vi "Data Manage Thread.vi"() -> ()   [LabVIEW 2016]
uses:
  <vilib>/Utility/error.llb/DialogType.ctl
  Architecture/Queue Management/ARC_Queue Create_Single.vi
  Architecture/Queue Management/ARC_Queue Valid.vi
  Architecture/Queue Management/ARC_Queue Insert Element.vi
  Architecture/Queue Management/ARC_Queue Remove Element.vi
  Architecture/Queue Management/ARC_Queue Destroy_Single.vi
panel:
  in  "Parameter":cluster{"Q-Local":string, "Variant":variant}
  out "Error Report":string
  out "Current State":string
  in  "Exit Program":bool
  in  "TempVariable":T1
  # "/* -------- Notes for All Users -------- */\nRecommand : \n[1].Display Setting Resolution -> 1440x900\n[2].Read Arch Notes First.\n[3].Make A Call When You Are In Trouble.\n\nTeam Members:\nPansino Soft,Pansino SDMA\n\nCopyright@2013 Pansino.Beijing\n\nVersion Number: 2013"
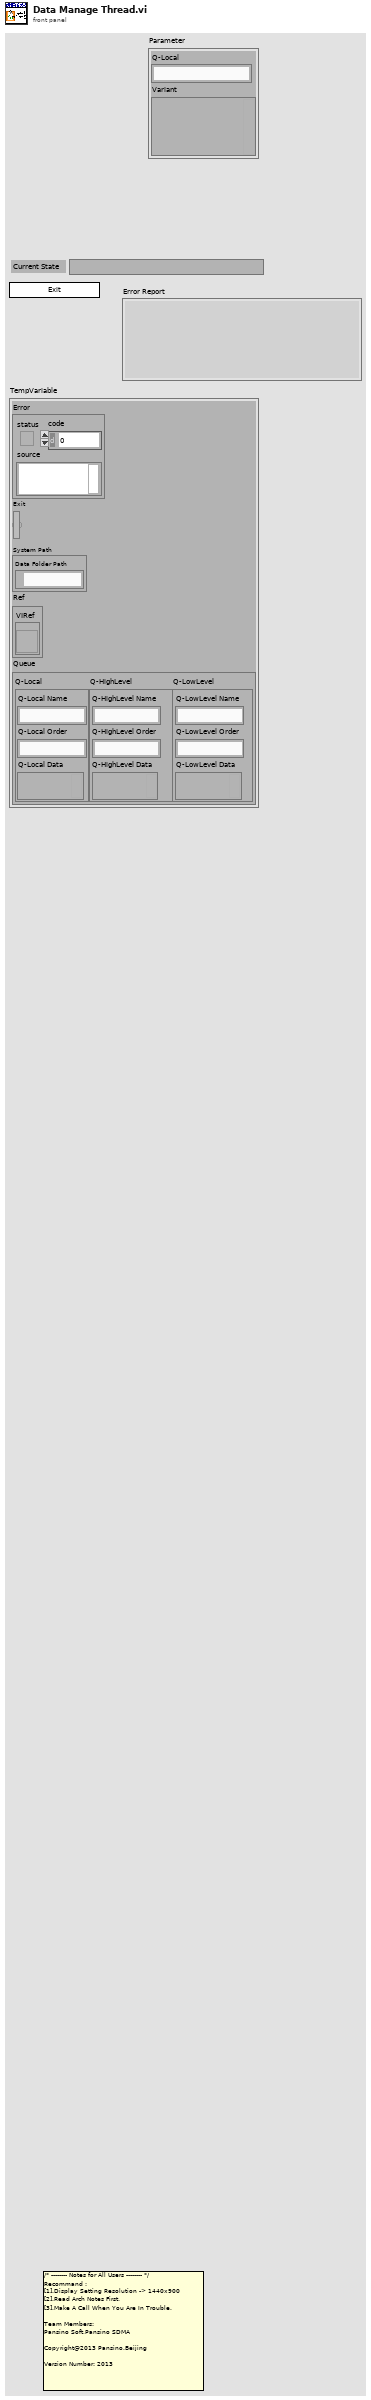
[diagram p1: front panel]
types:
  T1 = cluster{"Error":errorcluster, "Exit":bool, "System Path":cluster{"Data Folder Path":path}, "Ref":cluster{"VIRef":refnum<vi>}, "Queue":cluster{"Q-Local":cluster{"Q-Local Name":string, "Q-Local Order":string, "Q-Local Data":variant}, "Q-HighLevel":cluster{"Q-HighLevel Name":string, "Q-HighLevel Order":string, "Q-HighLevel Data":variant}, "Q-LowLevel":cluster{"Q-LowLevel Name":string, "Q-LowLevel Order":string, "Q-LowLevel Data":variant}}}
  T2 = typedef "DialogType.ctl" = u16
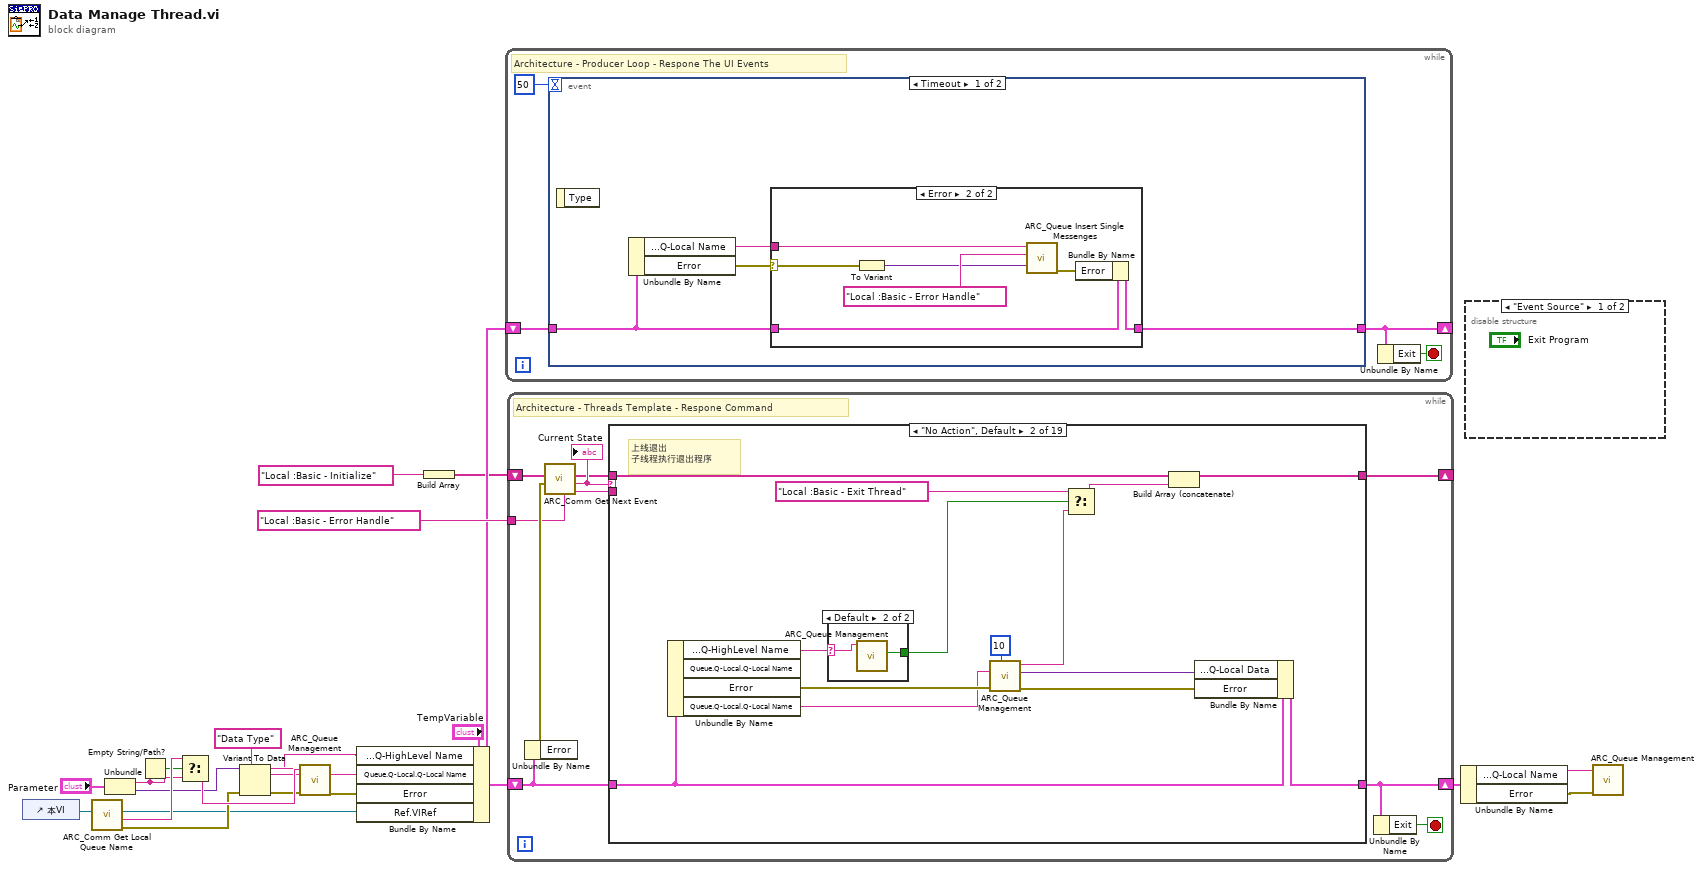
[diagram p0: block diagram]
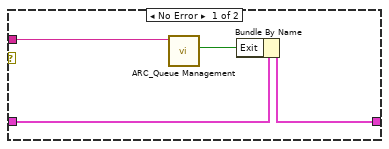
[diagram p2: hidden frame]
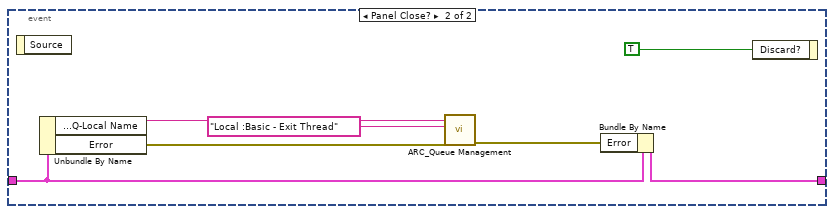
[diagram p3: hidden frame]
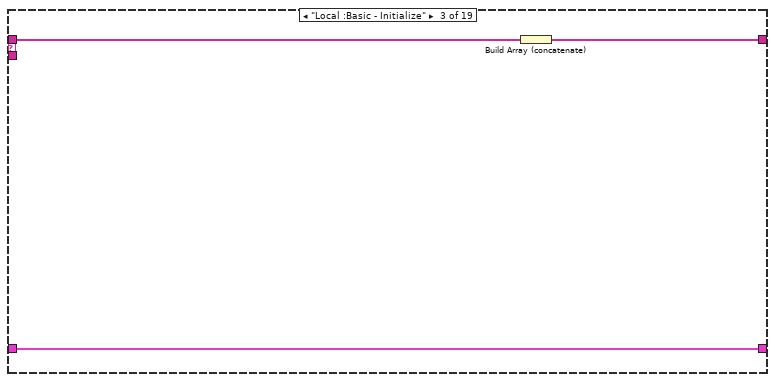
[diagram p7: hidden frame]
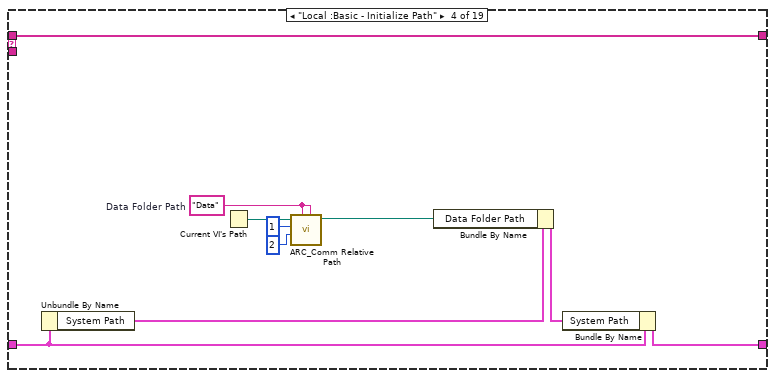
[diagram p8: hidden frame]
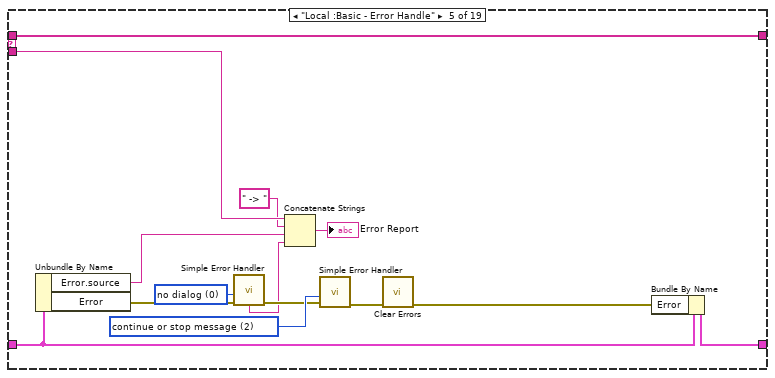
[diagram p9: hidden frame]
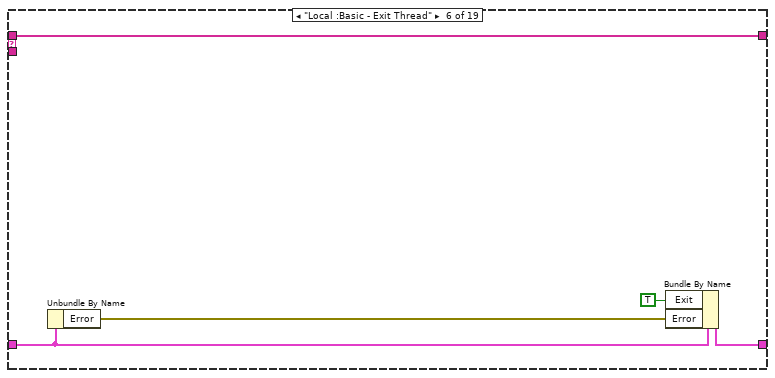
[diagram p10: hidden frame]
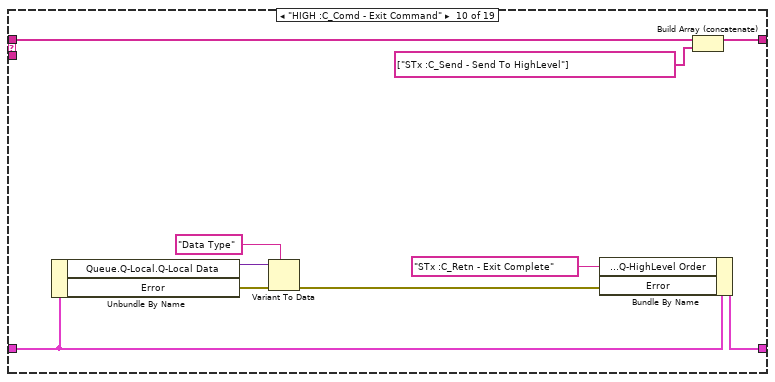
[diagram p14: hidden frame]
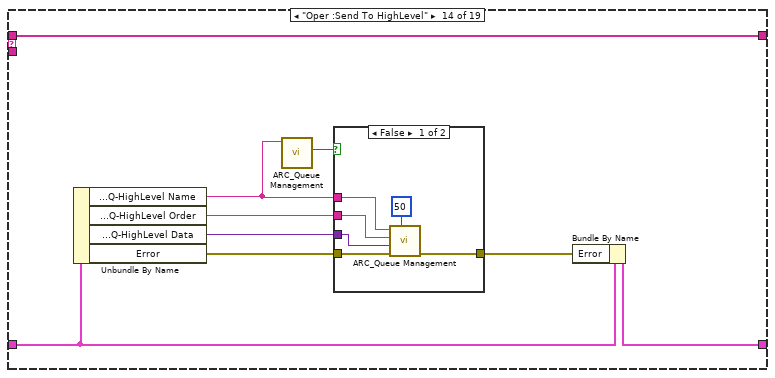
[diagram p18: hidden frame]
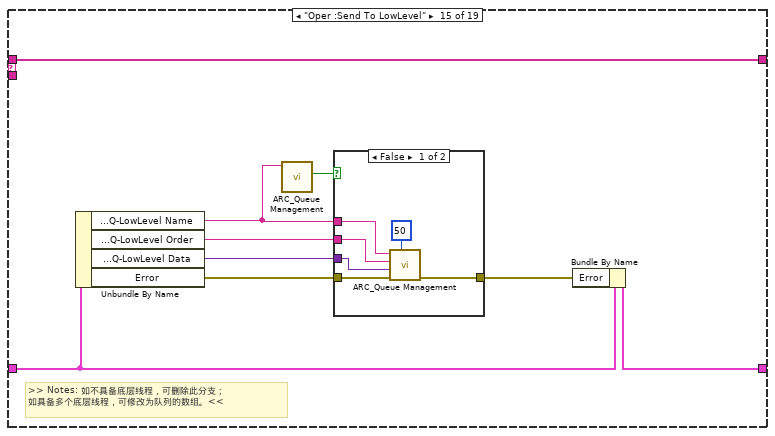
[diagram p20: hidden frame]
diagram:
  n1 = control-ref of="本VI"() -> (w7:refnum<vi>)
  n2 = call "ARC_Comm Get Local Queue Name.vi"("VI Ref"=w7) -> ("error out"=w8:errorcluster, "VI  Name"=w13:string, "VI Ref out"=w4:refnum<vi>)  [unwired: 8 in]
  n3 = Unbundle("Parameter") -> ("Q-Local"=w9:string, "Variant"=w12:variant)
  n4 = Empty String/Path?(string/path=w9) -> (empty?=w11:bool)
  n5 = Select(t=w13, s=w11, f=w9) -> (s? t:f=w14:string)
  n6 = Variant To Data(error in=w8, type="Data Type" ("Q-Command"), Variant=w12) -> (data=w1:string, error out=w6:errorcluster)
  n7 = call-poly "ARC_Queue Management.vi"("error in"=w6, "Queue Name"=w14) -> ("error out"=w3:errorcluster, "Queue Name dup"=w2:string)  [unwired: 7 in, 1 out]
  n8 = Bundle By Name(cluster="TempVariable", "Queue.Q-HighLevel.Q-HighLevel Name"=w1, "Queue.Q-Local.Q-Local Name"=w2, "Error"=w3, "Ref.VIRef"=w4) -> (w17:T1)
  n9 = Build Array("Local :Basic - Initialize") -> (w15:string[])
  n10 = while {
    shift-right: [w24] -> _
    shift-left: w17 -> [w25]
    stop <- w23 stop-if-true
    # "Architecture - Producer Loop - Respone The UI Events"
    n11 = event shown="[0] Timeout" {
      selector: _ -> [_ _]
      dyn-events: _ -> [_ _]
      timeout: 50 -> [_ _]
      tunnel: w25 -> [w29 w46]
      tunnel: [w30 w45] -> w24
      event Timeout {
        n12 = event-data() -> ()  [unwired: 1 in, 1 out]
        n13 = Unbundle By Name(w29) -> ("Queue.Q-Local.Q-Local Name"=w28:string, "Error"=w27:errorcluster)
        n14 = case shown="Error" w27 {
          selector: w27 -> [_ w41]
          tunnel: [w34 w39] -> w30
          tunnel: w29 -> [w32 w40]
          tunnel: w28 -> [w31 w38]
          frame No Error {
            n15 = call-poly "ARC_Queue Management.vi"("Queue Name(unamed)"=w31) -> ("Not Exist?"=w33:bool)  [unwired: 8 in, 2 out]
            n16 = Bundle By Name(cluster=w32, "Exit"=w33) -> (w34:T1)
          }
          frame Error {
            n17 = To Variant(anything=w41) -> (Variant=w36:variant)
            n18 = call "ARC_Queue Insert Single Messenges.vi"("Data"=w36, "Order"="Local :Basic - Error Handle" ("Event"), "Queue Name"=w38) -> ("error out"=w35:errorcluster)  [unwired: 8 in]
            n19 = Bundle By Name(cluster=w40, "Error"=w35) -> (w39:T1)
          }
        }
      }
      event Panel Close? {
        n20 = event-data() -> ()  [unwired: 1 in, 1 out]
        n21 = Unbundle By Name(w46) -> ("Queue.Q-Local.Q-Local Name"=w43:string, "Error"=w47:errorcluster)
        n22 = call-poly "ARC_Queue Management.vi"("error in (no error)"=w47, "Event"="Local :Basic - Exit Thread", "Queue Name(unamed)"=w43) -> ("error out"=w44:errorcluster)  [unwired: 7 in, 1 out]
        n23 = Bundle By Name(cluster=w46, "Error"=w44) -> (w45:T1)
        n24 = event-data("Discard?"=TRUE ("放弃？")) -> ()  [unwired: 1 in, 1 out]
      }
    }
    n25 = Unbundle By Name(w24) -> ("Exit"=w23:bool)
  }
  n26 = while {
    shift-right: [w52] -> w22
    shift-left: w17 -> [w54]
    shift-right: [w55] -> _
    shift-left: w15 -> [w58]
    tunnel: "Local :Basic - Error Handle" ("Error Handle") -> [w50]
    stop <- w51 stop-if-true
    # "Architecture - Threads Template - Respone Command"
    n27 = Unbundle By Name(w54) -> ("Error"=w53:errorcluster)
    n28 = call "ARC_Comm Get Next Event.vi"("Error Handle"=w50, "error in (no error)"=w53, "event queue in"=w58) -> ("prev event"=w49:string, "next event"=w57:string, "event queue out"=w56:string[])  [unwired: 3 in]
    "Current State" <- w57
    n29 = case shown="\"No Action\", Default" w57 {
      tunnel: w54 -> [w59 w74 w78 w87 w101 w105 w109 w111 w113 w121 w125 w127 w129 w136 w152 w163 w168 w175 w181]
      tunnel: w56 -> [w60 w67 w79 w89 w103 w108 w110 w112 w114 w124 w126 w128 w130 w139 w155 w164 w166 w176 w179]
      tunnel: [w60 w66 w77 w89 w103 w108 w110 w112 w114 w122 w126 w128 w130 w139 w155 w164 w165 w176 w178] -> w55
      tunnel: [w59 w73 w78 w88 w102 w106 w109 w111 w113 w123 w125 w127 w129 w135 w151 w163 w167 w174 w180] -> w52
      tunnel: w49 -> [_ _ _ _ w94 _ _ _ _ _ _ _ _ _ _ _ _ _ _]
      frame "----------Core Status----------" {
      }
      frame "No Action", Default {
        # "上线退出\n子线程执行退出程序"
        n30 = Unbundle By Name(w74) -> ("Queue.Q-HighLevel.Q-HighLevel Name"=w69:string, "Error"=w70:errorcluster, "Queue.Q-Local.Q-Local Name"=w68:string)  [unwired: 1 out]
        n31 = case shown="Default" w69 {
          selector: w69 -> [_ w75]
          tunnel: [_ w76] -> w64
          frame "" {
          }
          frame Default {
            n32 = call-poly "ARC_Queue Management.vi"("Queue Name(unamed)"=w75) -> ("Not Exist?"=w76:bool)  [unwired: 8 in, 2 out]
          }
        }
        n33 = call-poly "ARC_Queue Management.vi"("Time out(-1)_queue out"=10, "error in (no error)"=w70, "Queue Name(unamed)"=w68) -> ("error out"=w72:errorcluster, "Data"=w71:variant, "Event"=w62:string)  [unwired: 5 in, 1 out]
        n34 = Select(t="Local :Basic - Exit Thread" ("Event"), s=w64, f=w62) -> (s? t:f=w61:string)
        n35 = Build Array (concatenate)(w67, w61) -> (w66:string[])
        n36 = Bundle By Name(cluster=w74, "Queue.Q-Local.Q-Local Data"=w71, "Error"=w72) -> (w73:T1)
      }
      frame "Local :Basic - Initialize" {
        n37 = Build Array (concatenate)(w79) -> (w77:string[])
      }
      frame "Local :Basic - Initialize Path" {
        w82 = "Data"  # Data Folder Path
        n38 = Unbundle By Name(w87) -> ("System Path"=w81:cluster{"Data Folder Path":path})
        n39 = Current VI's Path() -> (path=w83:path)
        n40 = call "ARC_Comm Relative Path.vi"("Development Relative Path"=w82, "Run Time relative path"=w82, "Run-Time File Depth"=2, "Development File Depth"=1, "Root Path"=w83) -> ("Relative Path"=w86:path)  [unwired: 5 in, 1 out]
        n41 = Bundle By Name(cluster=w81, "Data Folder Path"=w86) -> (w80:cluster{"Data Folder Path":path})
        n42 = Bundle By Name(cluster=w87, "System Path"=w80) -> (w88:T1)
      }
      frame "Local :Basic - Error Handle" {
        w95 = T2 0 items=["no dialog", "OK message", "continue or stop message", "OK message + warnings", "continue/stop + warnings"] ("type of dialog (OK msg:1)")
        w98 = T2 2 items=["no dialog", "OK message", "continue or stop message", "OK message + warnings", "continue/stop + warnings"] ("type of dialog (OK msg:1)")
        n43 = Unbundle By Name(w101) -> ("Error.source"=w90:string, "Error"=w97:errorcluster)
        n44 = call <vilib>:"Simple Error Handler.vi"("type of dialog (OK msg:1)"=w95, "error in (no error)"=w97) -> ("error out"=w96:errorcluster, "message"=w92:string)  [unwired: 3 in, 3 out]
        n45 = Concatenate Strings(w94, " -> " ("字符串"), w90, w92) -> (→"Error Report":string)
        n46 = call <vilib>:"Simple Error Handler.vi"("type of dialog (OK msg:1)"=w98, "error in (no error)"=w96) -> ("error out"=w100:errorcluster)  [unwired: 3 in, 4 out]
        n47 = call <vilib>:"Clear Errors.vi"("error in (no error)"=w100) -> ("error out"=w99:errorcluster)  [unwired: 5 in, 1 out]
        n48 = Bundle By Name(cluster=w101, "Error"=w99) -> (w102:T1)
      }
      frame "Local :Basic - Exit Thread" {
        n49 = Unbundle By Name(w105) -> ("Error"=w107:errorcluster)
        n50 = Bundle By Name(cluster=w105, "Exit"=TRUE, "Error"=w107) -> (w106:T1)
      }
      frame "----------------Events--------------" {
      }
      frame "Event :" {
      }
      frame "----------Commond From HIGH----------" {
      }
      frame "HIGH :C_Comd - Exit Command" {
        n51 = Unbundle By Name(w121) -> ("Queue.Q-Local.Q-Local Data"=w120:variant, "Error"=w119:errorcluster)
        n52 = Variant To Data(error in=w119, type="Data Type" ("Data Type"), Variant=w120) -> (error out=w117:errorcluster)  [unwired: 1 out]
        n53 = Bundle By Name(cluster=w121, "Queue.Q-HighLevel.Q-HighLevel Order"="STx :C_Retn - Exit Complete" ("Data Type"), "Error"=w117) -> (w123:T1)
        n54 = Build Array (concatenate)(w124, string[] ["STx :C_Send - Send To HighLevel"] ("数组")) -> (w122:string[])
      }
      frame "----------Operation----------" {
      }
      frame "Oper :" {
      }
      frame "----------Communication----------" {
      }
      frame "Oper :Send To HighLevel" {
        n55 = Unbundle By Name(w136) -> ("Queue.Q-HighLevel.Q-HighLevel Name"=w138:string, "Queue.Q-HighLevel.Q-HighLevel Order"=w133:string, "Queue.Q-HighLevel.Q-HighLevel Data"=w132:variant, "Error"=w137:errorcluster)
        n56 = call-poly "ARC_Queue Management.vi"("Queue Name(unamed)"=w138) -> ("Not Exist?"=w134:bool)  [unwired: 8 in, 2 out]
        n57 = case shown="False" w134 {
          tunnel: w137 -> [w145 w146]
          tunnel: w138 -> [w143 _]
          tunnel: w133 -> [w141 _]
          tunnel: w132 -> [w142 _]
          tunnel: [w140 w146] -> w131
          frame False {
            n58 = call-poly "ARC_Queue Management.vi"("Time out(-1)_queue in"=50, "error in (no error)"=w145, "Data"=w142, "Event"=w141, "Queue Name(unamed)"=w143) -> ("error out"=w140:errorcluster)  [unwired: 5 in, 1 out]
          }
          frame True {
          }
        }
        n59 = Bundle By Name(cluster=w136, "Error"=w131) -> (w135:T1)
      }
      frame "Oper :Send To LowLevel" {
        # ">> Notes: 如不具备底层线程，可删除此分支；\n如具备多个底层线程，可修改为队列的数组。<<"
        n60 = Unbundle By Name(w152) -> ("Queue.Q-LowLevel.Q-LowLevel Name"=w154:string, "Queue.Q-LowLevel.Q-LowLevel Order"=w149:string, "Queue.Q-LowLevel.Q-LowLevel Data"=w148:variant, "Error"=w153:errorcluster)
        n61 = call-poly "ARC_Queue Management.vi"("Queue Name(unamed)"=w154) -> ("Not Exist?"=w150:bool)  [unwired: 8 in, 2 out]
        n62 = case shown="False" w150 {
          tunnel: w153 -> [w161 w162]
          tunnel: w154 -> [w159 _]
          tunnel: w149 -> [w157 _]
          tunnel: w148 -> [w158 _]
          tunnel: [w156 w162] -> w147
          frame False {
            n63 = call-poly "ARC_Queue Management.vi"("Time out(-1)_queue in"=50, "error in (no error)"=w161, "Data"=w158, "Event"=w157, "Queue Name(unamed)"=w159) -> ("error out"=w156:errorcluster)  [unwired: 5 in, 1 out]
          }
          frame True {
          }
        }
        n64 = Bundle By Name(cluster=w152, "Error"=w147) -> (w151:T1)
      }
      frame "----------Respond From LOW----------" {
      }
      frame "LOW :C_Resp - /* ADD NAME */" {
        n65 = Unbundle By Name(w168) -> ("Error"=w169:errorcluster)
        n66 = Build Array (concatenate)(w166) -> (w165:string[])
        n67 = Bundle By Name(cluster=w168, "Error"=w169) -> (w167:T1)
      }
      frame "LOW :C_Resp - /*Respond The Request*/" {
        n68 = Unbundle By Name(w175) -> ("Queue.Q-Local.Q-Local Data"=w172:variant, "Error"=w173:errorcluster)
        n69 = Variant To Data(error in=w173, type="Data Type" ("Data Type"), Variant=w172) -> (error out=w171:errorcluster)  [unwired: 1 out]
        n70 = Bundle By Name(cluster=w175, "Error"=w171) -> (w174:T1)
      }
      frame "LOW :C_Resp - Exit Complete" {
        # ">> Notes: 此处接收下层的返回指令；: 前代表下层的VI功能名，如ACTS等<<"
        n71 = Unbundle By Name(w181) -> ("Error"=w182:errorcluster)
        n72 = Build Array (concatenate)(w179, string[] ["STx :L_Core - Exit Thread"] ("数组")) -> (w178:string[])
        n73 = Bundle By Name(cluster=w181, "Error"=w182) -> (w180:T1)
      }
    }
    n74 = Unbundle By Name(w52) -> ("Exit"=w51:bool)
  }
  n75 = Unbundle By Name(w22) -> ("Queue.Q-Local.Q-Local Name"=w20:string, "Error"=w21:errorcluster)
  n76 = disable-structure shown="\"Event Source\"" {
    frame condition #0 (active) {
    }
    frame condition #1 {
    }
  }
  n77 = call-poly "ARC_Queue Management.vi"("error in (no error)"=w21, "Queue Name(unamed)"=w20) -> ()  [unwired: 7 in, 3 out]
